vi "Post-Install Custom Action.vi"(10 "Variant":variant) -> (0 "error out":errorcluster)   [LabVIEW 2020]
uses:
  <vilib>/Utility/traverseref.llb/TRef TravTarget.ctl
  <vilib>/Utility/traverseref.llb/VI Scripting - Traverse.lvlib
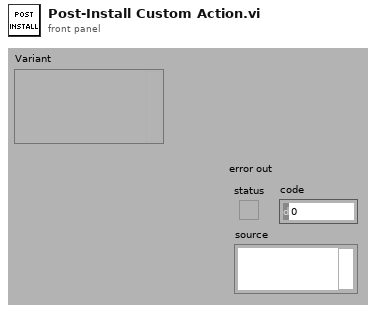
[diagram p1: front panel]
types:
  T1 = typedef "TRef TravTarget.ctl" = enum16{"FP", "BD", "Other"}
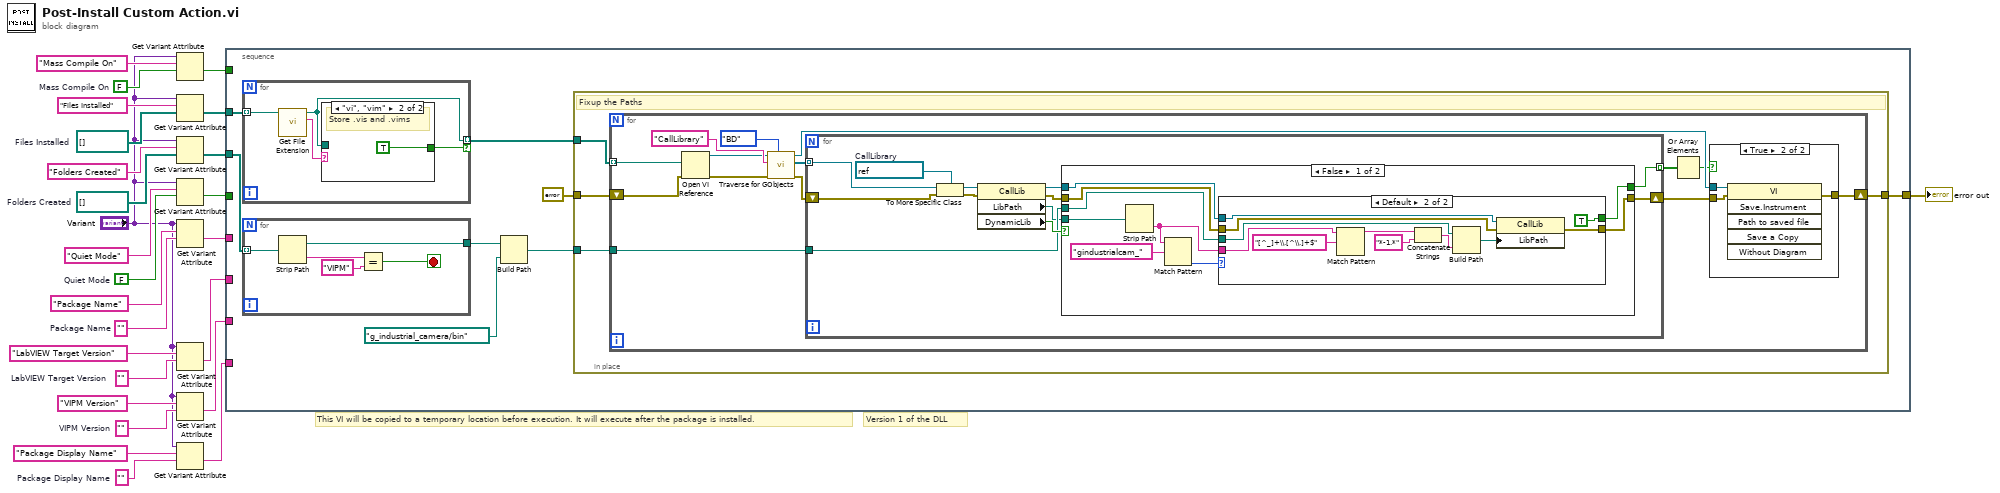
[diagram p0: block diagram]
diagram:
  w3 = path[] []  # Folders Created
  w4 = path[] []  # Files Installed
  w9 = FALSE  # Mass Compile On
  w10 = ""  # Package Display Name
  w17 = FALSE  # Quiet Mode
  w20 = ""  # VIPM Version
  w22 = ""  # LabVIEW Target Version
  w24 = ""  # Package Name
  # "Version 1 of the DLL"
  # "This VI will be copied to a temporary location before execution. It will execute after the package is installed."
  n1 = Get Variant Attribute(Variant="Variant", name="Mass Compile On", default value (empty Variant)=w9) -> (value=w11:bool)  [unwired: 1 in, 3 out]
  n2 = Get Variant Attribute(Variant="Variant", name="Files Installed", default value (empty Variant)=w4) -> (value=w6:path[])  [unwired: 1 in, 3 out]
  n3 = Get Variant Attribute(Variant="Variant", name="Folders Created", default value (empty Variant)=w3) -> (value=w7:path[])  [unwired: 1 in, 3 out]
  n4 = Get Variant Attribute(Variant="Variant", name="Quiet Mode", default value (empty Variant)=w17) -> (value=w12:bool)  [unwired: 1 in, 3 out]
  n5 = Get Variant Attribute(Variant="Variant", name="Package Name", default value (empty Variant)=w24) -> (value=w15:string)  [unwired: 1 in, 3 out]
  n6 = Get Variant Attribute(Variant="Variant", name="LabVIEW Target Version", default value (empty Variant)=w22) -> (value=w14:string)  [unwired: 1 in, 3 out]
  n7 = Get Variant Attribute(Variant="Variant", name="VIPM Version", default value (empty Variant)=w20) -> (value=w13:string)  [unwired: 1 in, 3 out]
  n8 = Get Variant Attribute(Variant="Variant", name="Package Display Name", default value (empty Variant)=w10) -> (value=w16:string)  [unwired: 1 in, 3 out]
  n9 = stacked-sequence {
    tunnel: w16 -> [_]
    tunnel: w15 -> [_]
    tunnel: w14 -> [_]
    tunnel: w13 -> [_]
    tunnel: w12 -> [_]
    tunnel: w11 -> [_]
    tunnel: w6 -> [w34]
    tunnel: w7 -> [w33]
    tunnel: [w29] -> w2
    frame #0 {
      n10 = for {
        tunnel: w34 -> [w43] mode=indexing
        tunnel: [w40] -> w32 mode=indexing if=w41
        n11 = call <vilib>:"Get File Extension.vi"("file"=w43) -> ("lowercase file extension"=w42:string, "dup file"=w40:path)  [unwired: 6 in, 3 out]
        n12 = case shown="\"vi\", \"vim\"" w42 {
          tunnel: [_ TRUE] -> w41
          tunnel: w40 -> [_ _]
          frame Default {
          }
          frame "vi", "vim" {
            # "Store .vis and .vims"
          }
        }
      }
      n13 = for {
        tunnel: w33 -> [w39] mode=indexing
        tunnel: [w38] -> w28
        stop <- w36 stop-if-true
        n14 = Strip Path(path=w39) -> (stripped path=w38:path, name=w37:string)
        n15 = Equal?(x=w37, y="VIPM") -> (x = y?=w36:bool)
      }
      n16 = Build Path(base path=w28, name or relative path=path "g_industrial_camera/bin") -> (appended path=w30:path)
      n17 = in-place {
        in-place-border: [w46] -> w29
        in-place-border: w32 -> [w48]
        in-place-border: errorcluster {"status"=FALSE, "code"=0, "source"=""} ("error in (no error)") -> [w47]
        in-place-border: w30 -> [w45]
        # "Fixup the Paths"
        n18 = for {
          tunnel: w48 -> [w60] mode=indexing
          shift-right: [w58] -> w46
          shift-left: w47 -> [w57]
          tunnel: w45 -> [w49]
          n19 = Open VI Reference(vi path=w60, error in (no error)=w57) -> (vi reference=w53:refnum<vi>, error out=w52:errorcluster)  [unwired: 4 in]
          n20 = call <vilib>:"Traverse for GObjects.vi"("Traverse Target"=TRef_TravTarget."BD", "error in (no error)"=w52, "Class Name"="CallLibrary", "VI Refnum"=w53) -> ("error out"=w56:errorcluster, "References"=w51:refnum<vi>[], "dup VI Refnum"=w62:refnum<vi>)  [unwired: 4 in, 1 out]
          n21 = for {
            tunnel: w51 -> [w67] mode=indexing
            shift-right: [w74] -> w61
            shift-left: w56 -> [w69]
            tunnel: [w65] -> w50 mode=indexing
            tunnel: w49 -> [w64]
            w68 = refnum<vi> refnum  # CallLibrary
            n22 = To More Specific Class(target class=w68, reference=w67, error in=w69) -> (specific class reference=w70:refnum<vi>, error out=w71:errorcluster)
            n23 = property class="CallLib"(reference=w70, error in=w71) -> (reference out=w73:refnum<vi>, error out=w72:errorcluster, "LibPath"=w63:path, "DynamicLib"=w66:bool)
            n24 = case shown="False" w66 {
              tunnel: [w83 w96] -> w74
              tunnel: w73 -> [w82 _]
              tunnel: w72 -> [w81 w96]
              tunnel: w63 -> [w79 _]
              tunnel: [w78 _] -> w65
              tunnel: w64 -> [w76 _]
              frame False {
                n25 = Strip Path(path=w79) -> (name=w75:string)  [unwired: 1 out]
                n26 = Match Pattern(string=w75, regular expression="gindustrialcam_") -> (offset past match=w77:i32)  [unwired: 1 in, 3 out]
                n27 = case shown="Default" w77 {
                  tunnel: [w84 w95] -> w83
                  tunnel: w82 -> [_ w93]
                  tunnel: w81 -> [w84 w92]
                  tunnel: [_ TRUE] -> w78
                  tunnel: w76 -> [_ w90]
                  tunnel: w75 -> [_ w86]
                  frame -1 {
                  }
                  frame Default {
                    n28 = Match Pattern(string=w86, regular expression="[^_]+\\.[^\\.]+$") -> (before substring=w89:string)  [unwired: 1 in, 3 out]
                    n29 = Concatenate Strings(w89, "*-1.*" ("string")) -> (w85:string)
                    n30 = Build Path(base path=w90, name or relative path=w85) -> (appended path=w94:path)
                    n31 = property class="CallLib"(reference=w93, error in=w92, "LibPath"=w94) -> (error out=w95:errorcluster)  [unwired: 1 out]
                  }
                }
              }
              frame True {
              }
            }
          }
          n32 = Or Array Elements(Boolean array=w50) -> (logical OR=w59:bool)
          n33 = case shown="True" w59 {
            tunnel: w62 -> [_ w99]
            tunnel: w61 -> [w97 w98]
            tunnel: [w97 w100] -> w58
            frame False {
            }
            frame True {
              n34 = invoke class="VI" method="Save.Instrument"(reference=w99, error in=w98) -> (error out=w100:errorcluster)  [unwired: 4 in, 5 out]
            }
          }
        }
      }
    }
  }
  "error out" <- w2
